vi "2DPseudoUniqueArraySet.vi"(8 "Colums":i32=6, 11 "Rows":i32=3) -> (0 "2D Double Array":i32[][](array[numeric]), 3 "2D String Array":string[][](array[string]))   [LabVIEW 2023]
uses:
  <vilib>/numeric/Random Number (Range) U64.vi
  <vilib>/numeric/sub_Random U32.vi
panel:
  # "Генерира 6 \"уникални\" числа.\n\"Унникалността\" се запазва единствено и само за елементите в колоните на даден ред,\n но не и между редовете."
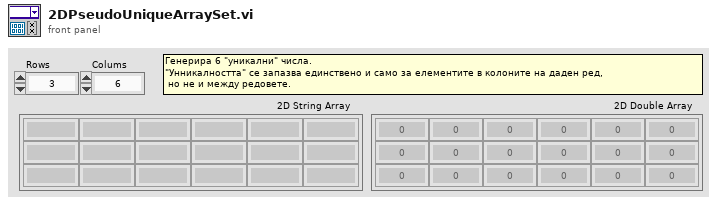
[diagram p1: front panel]
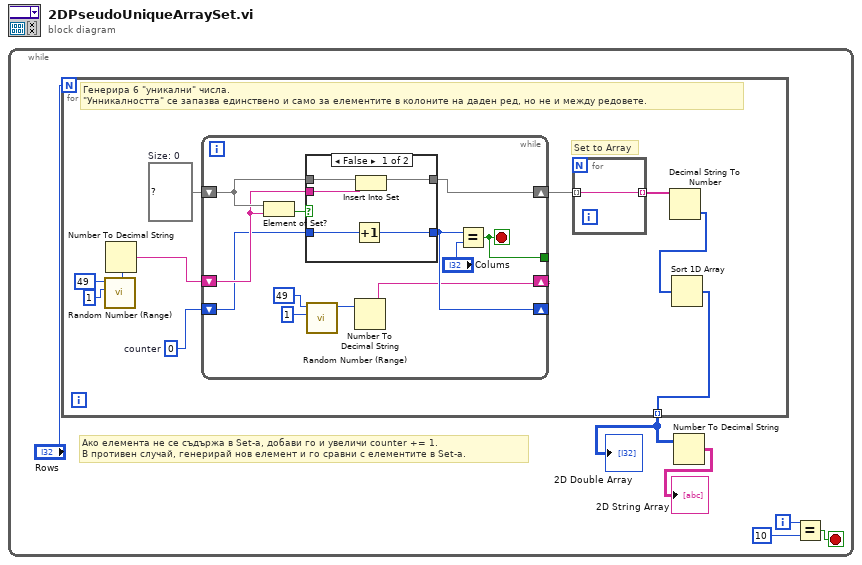
[diagram p0: block diagram]
diagram:
  n1 = while {
    i -> [w3]
    stop <- w1 stop-if-true
    # "Ако елемента не се съдържа в Set-а, добави го и увеличи counter += 1.\nВ противен случай, генерирай нов елемент и го сравни с елементите в Set-а."
    n2 = for {
      N: "Rows" -> [_]
      tunnel: [w9] -> w5 mode=indexing
      w10 = set{string} {}  # Size: 0
      w12 = 0  # counter
      # "Генерира 6 \"уникални\" числа.\n\"Унникалността\" се запазва единствено и само за елементите в колоните на даден ред, но не и между редовете."
      # "Set to Array"
      n3 = call-poly <vilib>:"Random Number (Range).vi"("lower bound (0)"=u64 1, "upper bound (100)"=u64 49) -> ("number"=w16:u64)  [unwired: 9 in]
      n4 = Number To Decimal String(number=w16) -> (decimal integer string=w13:string)  [unwired: 1 in]
      n5 = while {
        shift-right: [w26] -> w11
        shift-left: w10 -> [w28]
        shift-right: [w19] -> _
        shift-left: w13 -> [w27]
        shift-right: [w24] -> _
        shift-left: w12 -> [w25]
        tunnel: [w18] -> _
        stop <- w18 stop-if-true
        n6 = Element of Set?(10:w27, 11:w28) -> (3:w29:bool)
        n7 = case shown="False" w29 {
          tunnel: w28 -> [w34 w36]
          tunnel: w27 -> [w32 _]
          tunnel: [w33 w36] -> w26
          tunnel: w25 -> [w31 w35]
          tunnel: [w30 w35] -> w24
          frame False {
            n8 = Increment(x=w31) -> (x+1=w30:i32)
            n9 = Insert Into Set(10:w32, 11:w34) -> (3:w33:set{string})  [unwired: 1 out]
          }
          frame True {
          }
        }
        n10 = call-poly <vilib>:"Random Number (Range).vi"("lower bound (0)"=u64 1, "upper bound (100)"=u64 49) -> ("number"=w22:u64)  [unwired: 9 in]
        n11 = Number To Decimal String(number=w22) -> (decimal integer string=w19:string)  [unwired: 1 in]
        n12 = Equal?(x=w24, y="Colums") -> (x = y?=w18:bool)
      }
      n13 = for {
        tunnel: [w17] -> w8 mode=indexing
        tunnel: w11 -> [w17] mode=indexing
      }
      n14 = Decimal String To Number(string=w8) -> (number=w7:i32[])  [unwired: 2 in, 1 out]
      n15 = Sort 1D Array(array=w7) -> (sorted array=w9:i32[])
    }
    "2D Double Array" <- w5
    n16 = Number To Decimal String(number=w5) -> (decimal integer string=→"2D String Array":string[][])  [unwired: 1 in]
    n17 = Equal?(x=w3, y=10) -> (x = y?=w1:bool)
  }
